vi "ExpandTree__slk_tc.vi"(0 "tree control in":refnum<class "TreeControl.lvclass">, 11 "error in (no error)":errorcluster) -> (4 "tree control out":refnum<class "TreeControl.lvclass">, 15 "error out":errorcluster)   [LabVIEW 2020, in "TreeControl.lvclass"]
doc: "Expands the entire tree."
uses:
  Library/TreeControl.lvclass
  Library/TreeControl.lvclass/TreeControl.ctl
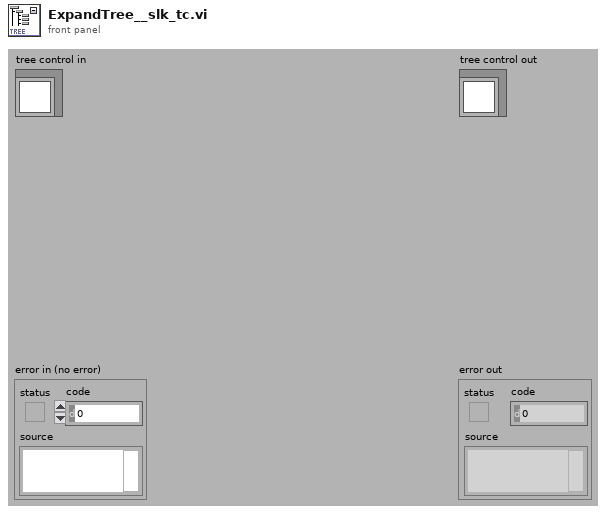
[diagram p1: front panel]
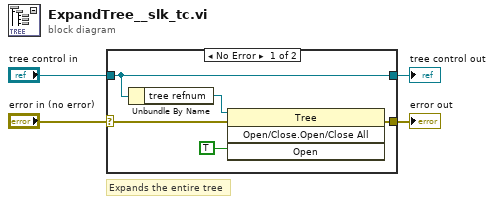
[diagram p0: block diagram]
diagram:
  # "Expands the entire tree"
  n1 = case shown="No Error" "error in (no error)" {
    selector: "error in (no error)" -> [w6 w11]
    tunnel: [w5 w11] -> w3
    tunnel: [w9 w10] -> w1
    tunnel: "tree control in" -> [w9 w10]
    frame No Error {
      n2 = Unbundle By Name(w9) -> ("tree refnum"=w8:refnum<vi>)
      n3 = invoke class="Tree" method="Open/Close.Open/Close All"(reference=w8, error in=w6, "Open"=TRUE ("Open?")) -> (error out=w5:errorcluster)  [unwired: 1 in, 3 out]
    }
    frame Error {
    }
  }
  "error out" <- w3
  "tree control out" <- w1
